vi "Measure.vi"(4 "error in (no error)":errorcluster, 5 "Method .NET Refnum":refnum<k24>, 6 "Live Curve Result Refnum":refnum<vi>, 7 "PalmSens in":refnum<class "PalmSens.lvclass">) -> (0 "error out":errorcluster, 1 "Time Stamp":timestamp, 2 "Curves":T1, 3 "PalmSens out":refnum<class "PalmSens.lvclass">)   [LabVIEW 2025, in "PalmSens.lvclass"]
uses:
  PalmSens.lvclass
  C:/Users/stef/code/palmsenssdk/labview/PalmSens/Libraries/PalmSens.Core.Simplified.LabVIEW.dll
  Libraries/PalmSens.Core.Simplified.LabVIEW.dll
  LiveCurveResult.ctl
  MeasurementResults.ctl
  PalmSens.lvclass/PalmSens.ctl
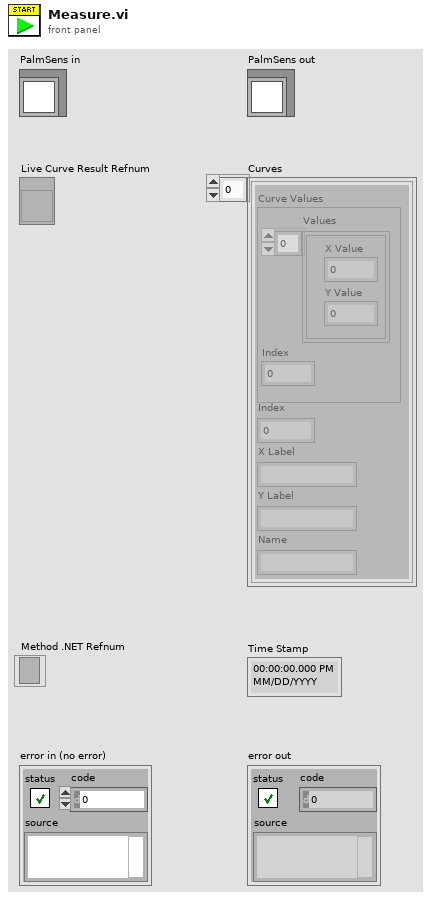
[diagram p1: front panel]
types:
  T1 = typedef "MeasurementResults.ctl" = T2[]
  T2 = typedef "LiveCurveResult.ctl" = cluster{"X Label":string, "Y Label":string, "Name":string, "Index":i16, "Curve Values":cluster{"Values":cluster{"X Value":dbl, "Y Value":dbl}[], "Index":i16}}
  T3 = typedef "ActiveMeasurementInfo.ctl" = cluster{"Active Measurement":refnum<k24>, "Is Measuring Refnum":refnum<vi>, "Live Curve Result Refnum":refnum<vi>}
  T4 = typedef "MeasurementsResult.ctl" = cluster{"Name":string, "Curves":T1, "Index":i32}[]
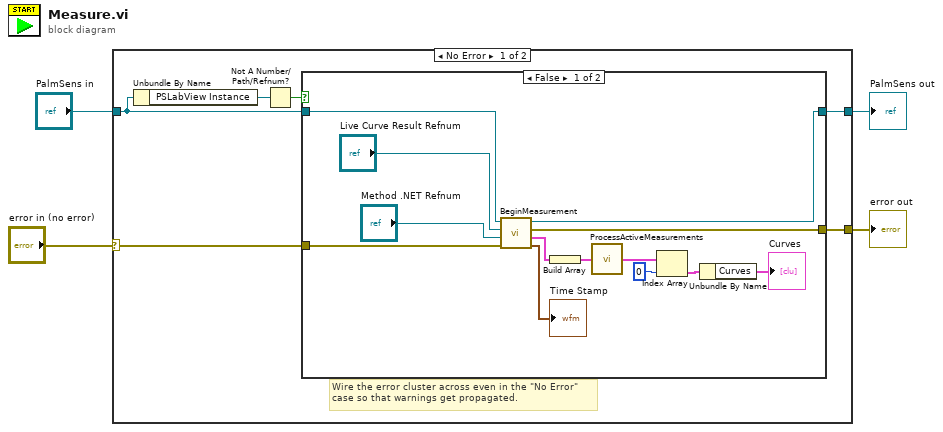
[diagram p0: block diagram]
diagram:
  n1 = case shown="No Error" "error in (no error)" {
    selector: "error in (no error)" -> [w8 w27]
    tunnel: [w7 w27] -> w3
    tunnel: [w6 w26] -> w1
    tunnel: "PalmSens in" -> [w5 w26]
    frame No Error {
      # "Wire the error cluster across even in the \"No Error\"\ncase so that warnings get propagated."
      n2 = Unbundle By Name(w5) -> ("PSLabView Instance"=w9:refnum<k24>)
      n3 = Not A Number/Path/Refnum?(number/path/refnum=w9) -> (NaN/Path/Refnum?=w10:bool)
      n4 = case shown="False" w10 {
        tunnel: w8 -> [w21 w25]
        tunnel: [w19 w25] -> w7
        tunnel: w5 -> [w20 w24]
        tunnel: [w18 w24] -> w6
        frame False {
          n5 = call-dynamic "BeginMeasurement.vi"("error in (no error)"=w21, "Method .NET Refnum"="Method .NET Refnum", "Live Curve Result Refnum"="Live Curve Result Refnum", "PalmSens in"=w20) -> ("Time Stamp"=→"Time Stamp":timestamp, "Active Measurement Info"=w22:T3, "error out"=w19:errorcluster, "PalmSens out"=w18:refnum<class "PalmSens.lvclass">)
          n6 = Build Array(w22) -> (w23:T3[])
          n7 = call "ProcessActiveMeasurements.vi"("Active Measurements"=w23) -> ("Measurements"=w17:T4)
          n8 = Index Array(array=w17, index=0) -> (element=w15:cluster{"Name":string, "Curves":T1, "Index":i32})
          n9 = Unbundle By Name(w15) -> ("Curves"=→"Curves":T1)
        }
        frame True {
        }
      }
    }
    frame Error {
    }
  }
  "error out" <- w3
  "PalmSens out" <- w1
